vi "BitfileDownloadedBroadcast_Name.vi"() -> (1 "message name":string="FpgaBitfileManager.BitfileDownloaded")   [LabVIEW 2017, in "FpgaBitfileManager.lvlib"]
uses:
  <vilib>/addons/InsightCM/Devices/Shared/Common/FpgaBitfileManager/FpgaBitfileManager.lvlib
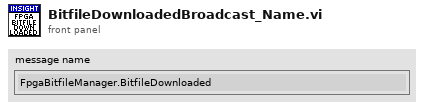
[diagram p1: front panel]
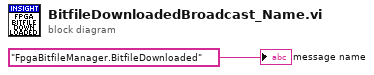
[diagram p0: block diagram]
diagram:
  "message name" <- "FpgaBitfileManager.BitfileDownloaded" ("ProcessName")
